vi "NewtonsPSM_Retrieve_Sweep_LCR.vi"(0 "VISA session":refnum<visa-resource-name>, 11 "error in (no error)":errorcluster) -> (1 "Q Factor":cluster{dbl[], dbl[]}(graph), 2 "Tan d":cluster{dbl[], dbl[]}(graph), 3 "Impedance":cluster{dbl[], dbl[]}(graph), 4 "dup VISA session":refnum<visa-resource-name>, 6 "Read Strings":string, 8 "Nb of points":dbl, 10 "Resistance R":cluster{dbl[], dbl[]}(graph), 12 "Phase":cluster{dbl[], dbl[]}(graph), 13 "Inductance L":cluster{dbl[], dbl[]}(graph), 14 "Capacitance C":cluster{dbl[], dbl[]}(graph), 15 "error out":errorcluster)   [LabVIEW 2025, in "NewtonsPSM1735.lvlib"]
doc: "This VI readback the Datastores into the PPA2530."
uses:
  NewtonsPSM1735.lvlib
panel:
  out "Retrieving Finished":bool
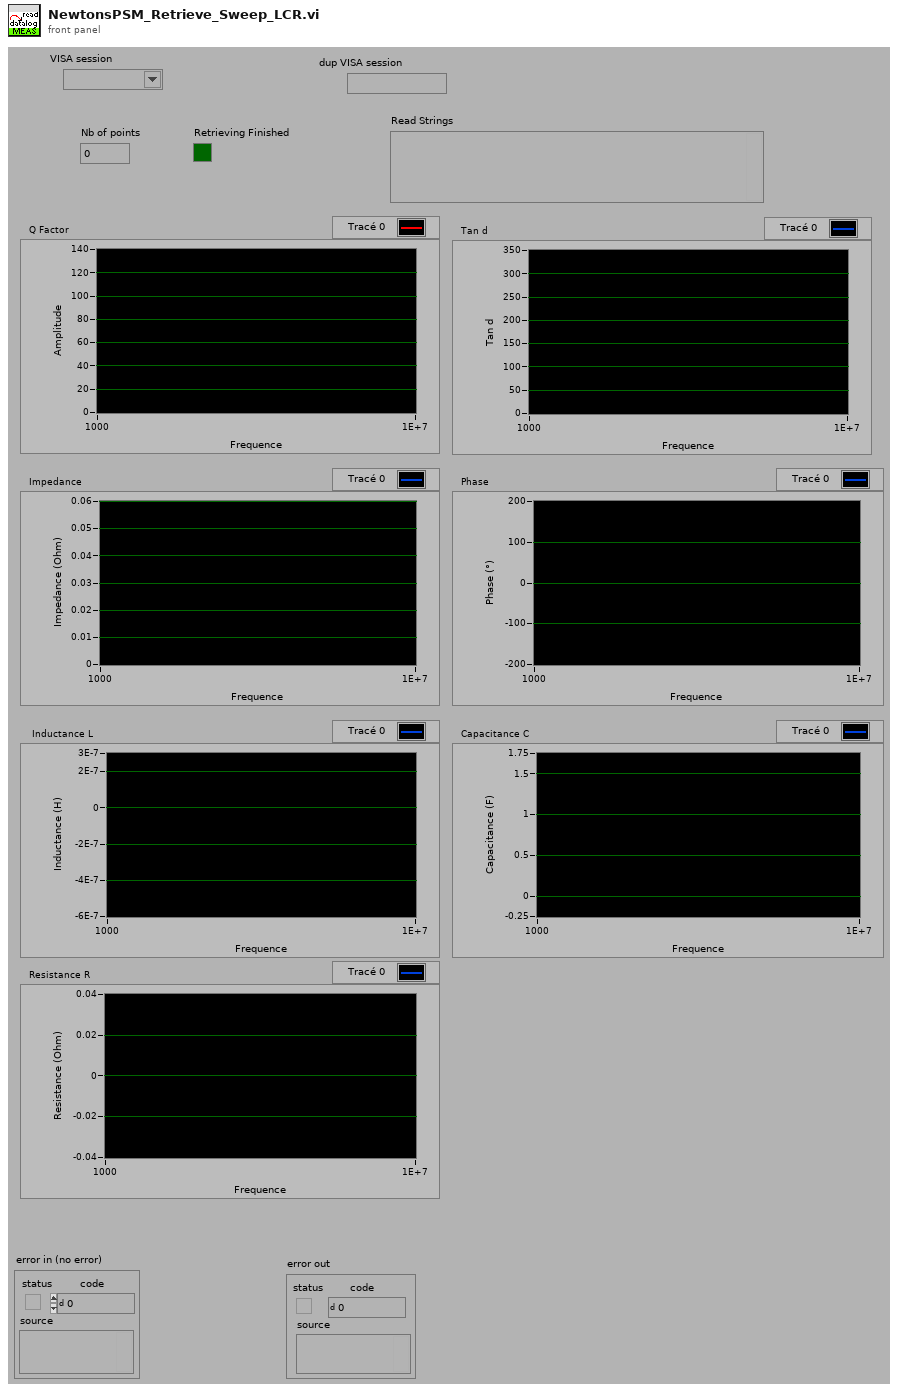
[diagram p1: front panel]
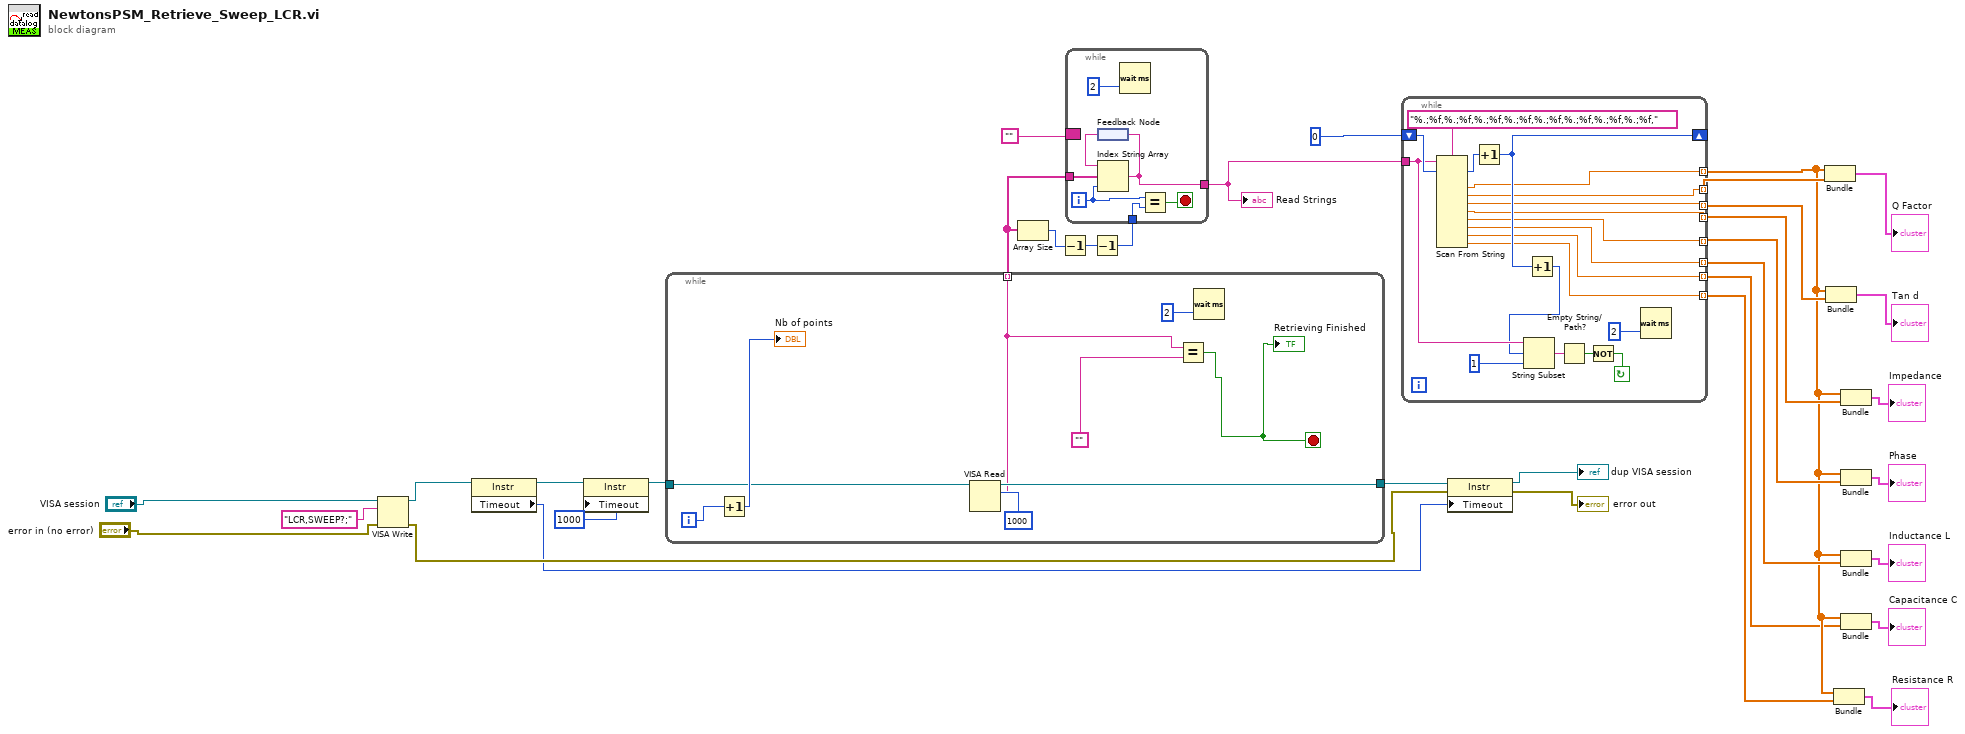
[diagram p0: block diagram]
diagram:
  n1 = VISA Write(VISA resource name="VISA session", write buffer="LCR,SWEEP?;" ("buffer à écrire"), error in (no error)="error in (no error)") -> (VISA resource name out=w3:refnum<visa-resource-name>, error out=w6:errorcluster)  [unwired: 1 out]
  n2 = property class="Instr"(reference=w3) -> (reference out=w4:refnum<visa-resource-name>, "Timeout"=w2:u32)  [unwired: 1 in, 1 out]
  n3 = property class="Instr"(reference=w4, "Timeout"=u32 1000 ("General Settings:Timeout Value")) -> (reference out=w10:refnum<visa-resource-name>)  [unwired: 1 in, 1 out]
  n4 = while {
    tunnel: [w41] -> w9
    tunnel: [w39] -> w33 mode=indexing
    tunnel: w10 -> [w37]
    i -> [w42]
    stop <- w36 stop-if-true
    n5 = Increment(x=w42) -> (x+1=→"Nb of points":i32)
    n6 = VISA Read(VISA resource name=w37, byte count=u32 1000 ("ÊÞ²Ä¶³ÝÄi0j")) -> (VISA resource name out=w41:refnum<visa-resource-name>, read buffer=w39:string)  [unwired: 1 in, 2 out]
    n7 = Equal?(x=w39, y="") -> (x = y?=w36:bool)
    "Retrieving Finished" <- w36
    n8 = Wait (ms)(milliseconds to wait=u32 2 ("attente (ms)")) -> ()  [unwired: 1 out]
  }
  n9 = Array Size(array=w33) -> (size(s)=w31:i32)
  n10 = Decrement(x=w31) -> (x-1=w30:i32)
  n11 = Decrement(x=w30) -> (x-1=w29:i32)
  n12 = while {
    tunnel: w33 -> [w50]
    tunnel: [w48] -> w32
    tunnel: w29 -> [w46]
    border: "" -> [_]
    i -> [w47]
    stop <- w49 stop-if-true
    n13 = feedback #1() -> (w45:string)
    n14 = Index String Array(1:w47, 2:w50, 3:w45) -> (0:w48:string)
    n15 = feedback-in #1(w48) -> ()
    n16 = Wait (ms)(milliseconds to wait=u32 2 ("attente (ms)")) -> ()  [unwired: 1 out]
    n17 = Equal?(x=w47, y=w46) -> (x = y?=w49:bool)
  }
  "Read Strings" <- w32
  n18 = while {
    shift-left: 0 -> [w63]
    shift-right: [w61] -> _
    tunnel: [w57] -> w23 mode=indexing
    tunnel: w32 -> [w62]
    tunnel: [w58] -> w25 mode=indexing
    tunnel: [w59] -> w17 mode=indexing
    tunnel: [w56] -> w20 mode=indexing
    tunnel: [w55] -> w19 mode=indexing
    tunnel: [w54] -> w18 mode=indexing
    tunnel: [w53] -> w16 mode=indexing
    tunnel: [w52] -> w15 mode=indexing
    stop <- w66 continue-if-true
    n19 = Scan From String(format string="%.;%f,%.;%f,%.;%f,%.;%f,%.;%f,%.;%f,%.;%f,%.;%f,", input string=w62, initial scan location=w63) -> (offset past scan=w64:u32, output 1=w59:dbl, output 2=w58:dbl, output 3=w57:dbl, output 4=w56:dbl, output 5=w55:dbl, output 6=w54:dbl, output 7=w53:dbl, output 8=w52:dbl)  [unwired: 1 in, 10 out]
    n20 = Increment(x=w64) -> (x+1=w61:u32)
    n21 = Increment(x=w61) -> (x+1=w60:u32)
    n22 = String Subset(string=w62, offset (0)=w60, length (rest)=1) -> (substring=w68:string)
    n23 = Empty String/Path?(string/path=w68) -> (empty?=w67:bool)
    n24 = Not(x=w67) -> (.not. x?=w66:bool)
    n25 = Wait (ms)(milliseconds to wait=u32 2 ("attente (ms)")) -> ()  [unwired: 1 out]
  }
  n26 = property class="Instr"(reference=w9, error in=w6, "Timeout"=w2) -> (reference out=→"dup VISA session":refnum<visa-resource-name>, error out=→"error out":errorcluster)
  n27 = Bundle(w17, w25) -> (→"Q Factor":cluster{dbl[], dbl[]})  [unwired: 1 out]
  n28 = Bundle(w17, w23) -> (→"Tan d":cluster{dbl[], dbl[]})  [unwired: 1 out]
  n29 = Bundle(w17, w15) -> (→"Resistance R":cluster{dbl[], dbl[]})  [unwired: 1 out]
  n30 = Bundle(w17, w20) -> (→"Impedance":cluster{dbl[], dbl[]})  [unwired: 1 out]
  n31 = Bundle(w17, w19) -> (→"Phase":cluster{dbl[], dbl[]})  [unwired: 1 out]
  n32 = Bundle(w17, w18) -> (→"Inductance L":cluster{dbl[], dbl[]})  [unwired: 1 out]
  n33 = Bundle(w17, w16) -> (→"Capacitance C":cluster{dbl[], dbl[]})  [unwired: 1 out]
